vi "parseError.vi"(7 "depth":i32=1, 8 "error in (no error)":errorcluster, 10 "extended error info":string, 11 "status code":i32) -> (0 "error out":errorcluster)   [LabVIEW 2020, in "box.lvlib"]
uses:
  box.lvlib
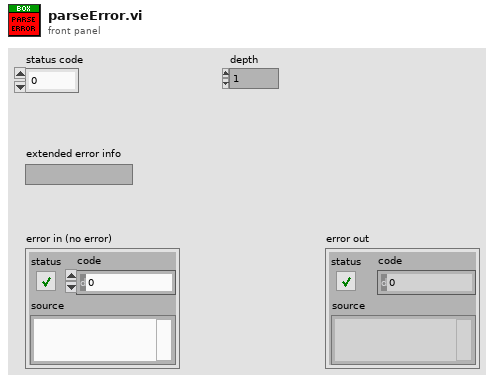
[diagram p1: front panel]
types:
  T1 = cluster{"status":bool, "status code":i32, string}
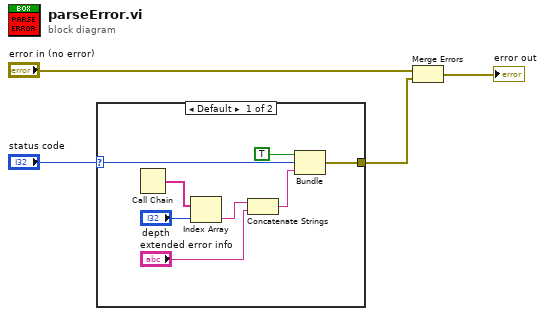
[diagram p0: block diagram]
diagram:
  n1 = case shown="Default" "status code" {
    selector: "status code" -> [w7 _]
    tunnel: [w6 _] -> w2
    frame Default {
      n2 = Call Chain() -> (call chain=w10:string[])
      n3 = Index Array(array=w10, index="depth") -> (element=w8:string)
      n4 = Concatenate Strings(w8, "extended error info") -> (w12:string)
      n5 = Bundle("status"=TRUE, "status code"=w7, w12) -> (w6:T1)  [unwired: 1 out]
    }
    frame 0 {
    }
  }
  n6 = Merge Errors("error in (no error)", w2) -> (→"error out":errorcluster)
